vi "Menu Button Pressed.vi"(8 "error in (no error)":errorcluster, 10 "Menu Reference":refnum<vi>, 11 "Menu Items In":refnum<class "MenuButton.lvclass">[](array[class])) -> (0 "error out":errorcluster, 3 "Menu Items Out":refnum<class "MenuButton.lvclass">[](array[class]))   [LabVIEW 2017, in "MenuButtons.lvlib" / "MenuButton Event Handler.lvclass"]
uses:
  MenuButton Event Handler.lvclass
  MenuButton/MenuButton.lvclass
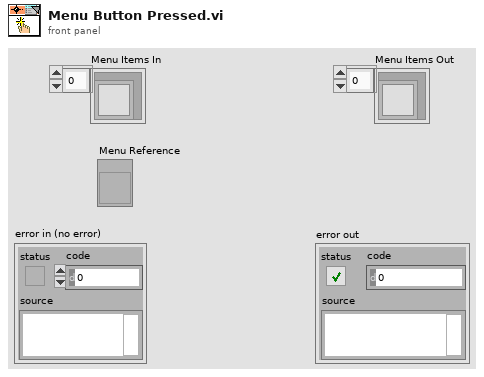
[diagram p1: front panel]
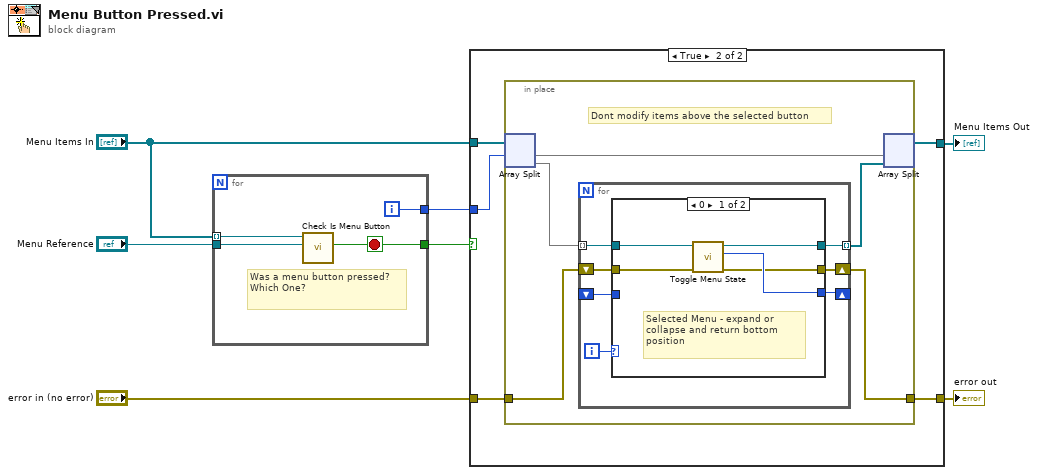
[diagram p0: block diagram]
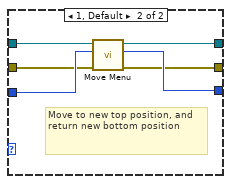
[diagram p3: hidden frame]
diagram:
  n1 = for {
    tunnel: "Menu Items In" -> [w11] mode=indexing
    tunnel: "Menu Reference" -> [w10]
    tunnel: [w9] -> w5
    tunnel: [w8] -> w4
    i -> [w8]
    stop <- w9 stop-if-true
    # "Was a menu button pressed? Which One?"
    n2 = call "Check Is Menu Button.vi"("Menu Reference"=w10, "MenuButton in"=w11) -> ("Is this Menu Button?"=w9:bool)  [unwired: 8 in, 1 out]
  }
  n3 = case shown="True" w5 {
    tunnel: "Menu Items In" -> [w13 w18]
    tunnel: w4 -> [_ w17]
    tunnel: [w13 w16] -> w3
    tunnel: "error in (no error)" -> [w12 w15]
    tunnel: [w12 w14] -> w1
    frame False {
    }
    frame True {
      n4 = in-place {
        in-place-border: w15 -> [w20]
        in-place-border: [w19] -> w14
        # "Dont modify items above the selected button"
        n5 = in-place-split #1(w18, w17) -> (w23:refnum<class "MenuButton.lvclass">[], w22:refnum<class "MenuButton.lvclass">[])
        n6 = for {
          tunnel: w22 -> [w29] mode=indexing
          tunnel: [w28] -> w21 mode=indexing
          shift-right: [w27] -> _
          shift-left: _ -> [w26]
          shift-right: [w24] -> w19
          shift-left: w20 -> [w25]
          i -> [w30]
          n7 = case shown="0" w30 {
            tunnel: w29 -> [w35 w41]
            tunnel: [w34 w40] -> w28
            tunnel: [w33 w38] -> w27
            tunnel: w26 -> [_ w39]
            tunnel: w25 -> [w32 w37]
            tunnel: [w31 w36] -> w24
            frame 0 {
              # "Selected Menu - expand or collapse and return bottom position"
              n8 = call "Toggle Menu State.vi"("error in (no error)"=w32, "MenuButton in"=w35) -> ("error out"=w31:errorcluster, "Menu Bottom Position"=w33:u32, "MenuButton out"=w34:refnum<class "MenuButton.lvclass">)  [unwired: 7 in]
            }
            frame 1, Default {
              # "Move to new top position, and return new bottom position"
              n9 = call "Move Menu.vi"("error in (no error)"=w37, "Starting Top Position"=w39, "MenuButton in"=w41) -> ("error out"=w36:errorcluster, "Ending Bottom Position"=w38:i32, "MenuButton out"=w40:refnum<class "MenuButton.lvclass">)  [unwired: 6 in]
            }
          }
        }
        n10 = in-place-split #1(w23, w21) -> (w16:refnum<class "MenuButton.lvclass">[])  [unwired: 1 out]
      }
    }
  }
  "Menu Items Out" <- w3
  "error out" <- w1
